vi "Plot init properties.vi"(5 "First call? (init)":bool, 7 "# plots":i32=2, 8 "error in (no error)":errorcluster, 11 "Refs":T1) -> (0 "error out":errorcluster, 3 "Refs (dup)":T1)   [LabVIEW 2021, in "RocketPlot.lvlib"]
uses:
  RocketPlot.lvlib
  TypeDefs/Plot UI references.ctl
  Classes/RocketPlotHandle/RocketPlotHandle.lvclass
  <userlib>/bjustice/TipStripOOPanel/Classes/TipPanelHandle/TipPanelHandle.lvclass
  TypeDefs/Plot top row.ctl
  TypeDefs/plot load data V2.ctl
  TypeDefs/plot properties V2.ctl
  TypeDefs/plot attributes V2.ctl
  TypeDefs/Plot scale axis properties.ctl
  TypeDefs/Plot general properties.ctl
  <vilib>/Utility/miscctls.llb/LVPositionTypeDef.ctl
  <vilib>/Utility/miscctls.llb/LVPointTypeDef.ctl
  <vilib>/Utility/colorconv.llb/RGB to Color.vi
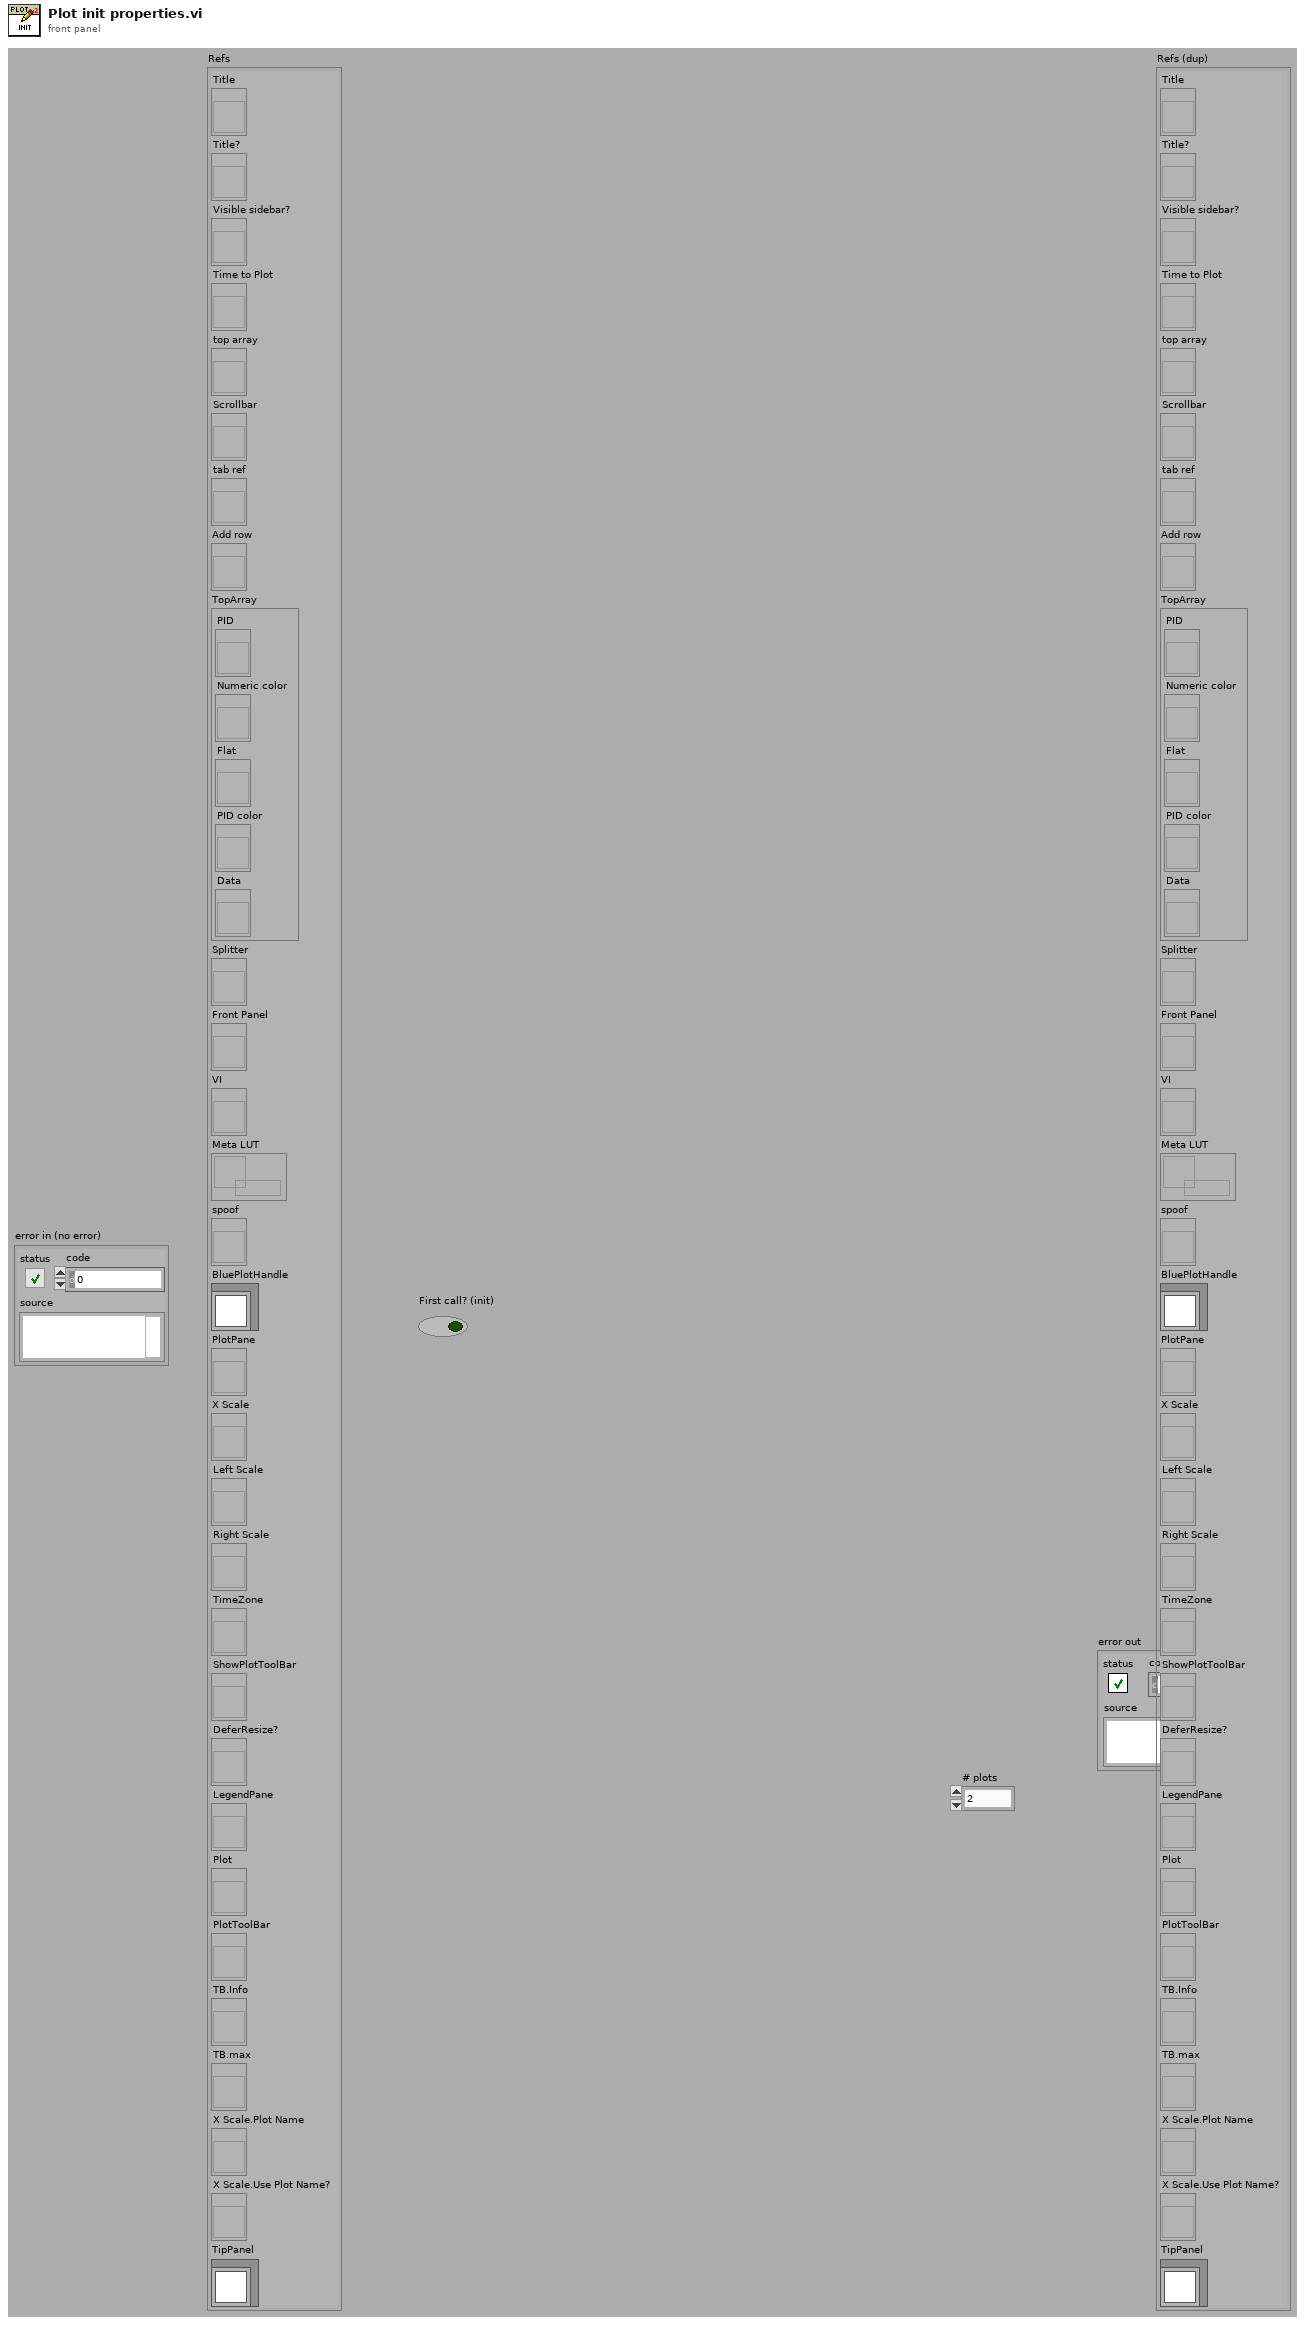
[diagram p1: front panel]
types:
  T1 = typedef "RocketPlot.lvlib/Plot UI references.ctl" = cluster{"Title":refnum<vi>, "Title?":refnum<vi>, "Visible sidebar?":refnum<vi>, "Time to Plot":refnum<vi>, "top array":refnum<vi>, "Scrollbar":refnum<vi>, "tab ref":refnum<vi>, "Add row":refnum<vi>, "TopArray":cluster{"PID":refnum<vi>, "Numeric color":refnum<vi>, "Flat":refnum<vi>, "PID color":refnum<vi>, "Data":refnum<vi>}, "Splitter":refnum<vi>, "Front Panel":refnum<vi>, "VI":refnum<vi>, "Meta LUT":refnum<data-value>, "spoof":refnum<vi>, "BluePlotHandle":refnum<class "RocketPlotHandle.lvclass">, "PlotPane":refnum<vi>, "X Scale":refnum<vi>, "Left Scale":refnum<vi>, "Right Scale":refnum<vi>, "TimeZone":refnum<vi>, "ShowPlotToolBar":refnum<vi>, "DeferResize?":refnum<vi>, "LegendPane":refnum<vi>, "Plot":refnum<vi>, "PlotToolBar":refnum<vi>, "TB.Info":refnum<vi>, "TB.max":refnum<vi>, "X Scale.Plot Name":refnum<vi>, "X Scale.Use Plot Name?":refnum<vi>, "TipPanel":refnum<class "TipPanelHandle.lvclass">}
  T2 = typedef "RocketPlot.lvlib/plot load data V2.ctl" = cluster{"plots":T3[], "X-axis":T5, "Y-axes":T5[], "General":T6}
  T3 = typedef "RocketPlot.lvlib/plot properties V2.ctl" = cluster{"attributes":T4, "Numeric":dbl, "Flatline?":bool}
  T4 = typedef "RocketPlot.lvlib/plot attributes V2.ctl" = cluster{"Plot Color":u32, "Point Style":u8, "Line Style":u8, "Plot Interpolation":u8, "Line Width":u8, "Bar Plot Style":u8, "Fill To":i16, "X Scale Index":u32, "Y Scale Index":u32, "Anti-aliased":bool, "Label Format":u8, "Digital Transition Type":u8, "Digital Transition Location":u8, "Digital Line Style":u8, "Fill/Point Color":u32, "Plot Name":string, "Visible":bool}
  T5 = typedef "RocketPlot.lvlib/Plot scale axis properties.ctl" = cluster{"Name Label.Text":string, "Style":u8, "Tick Colors:Minor Tick Color":u32, "Tick Colors:Tick Color":u32, "Marker Colors:Text Color":u32, "Grid Colors:Major Color":u32, "Grid Colors:Minor Color":u32, "Mapping Mode":u8, "Flipped":bool, "Name Label.Visible":bool, "Name Label.Text Colors:Text Color":u32, "Scale Fit":u8, "Range:Maximum":dbl, "Range:Minimum":dbl, "Offset and Multiplier:Multiplier":dbl, "Offset and Multiplier:Offset":dbl, "Name Label.Font:Size":u32, "Marker.Font:Size":u32, "Uniform Marker Spacing?":bool, "Format String":string}
  T6 = typedef "RocketPlot.lvlib/Plot general properties.ctl" = cluster{"Title":string, "Time to Plot":dbl, "Title.Visible":bool, "Sidebar.Visible":bool, "Plot Area:Colors:BG Color":u32, "X Scale.Plot Name":string, "X Scale.Use Plot Name":bool}
  T7 = typedef "LVPointTypeDef.ctl" = cluster{"Horizontal":i16, "Vertical":i16}
  T8 = typedef "LVPositionTypeDef.ctl" = cluster{"Left":i32, "Top":i32}
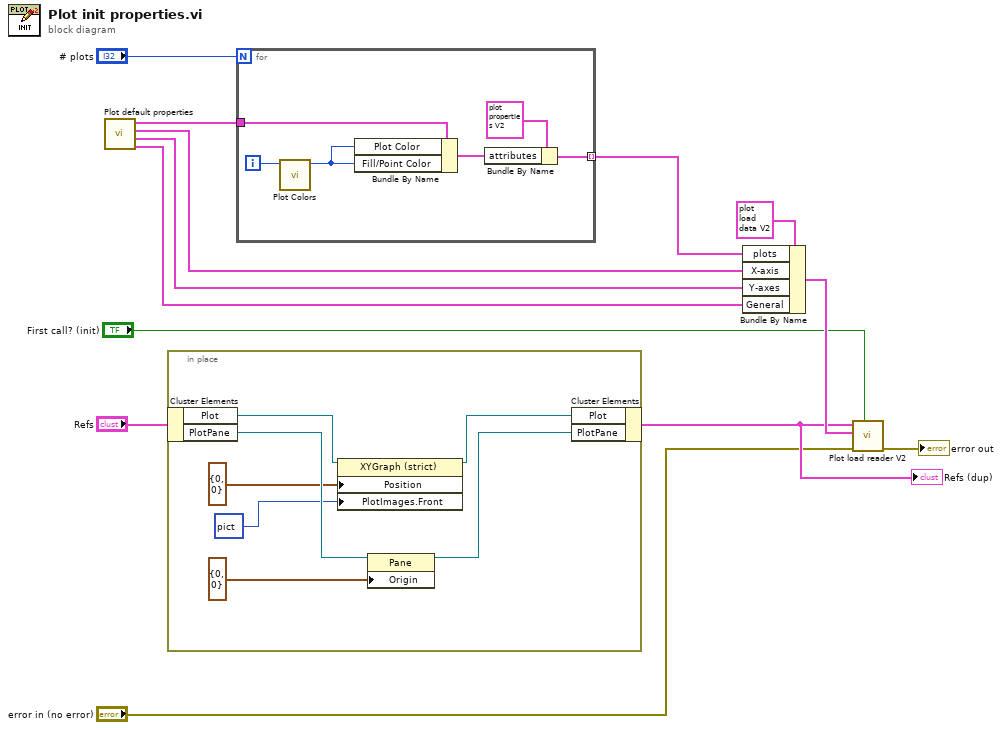
[diagram p0: block diagram]
diagram:
  n1 = call "Plot default properties.vi"() -> ("General"=w12:T6, "Default Y-axes"=w11:T5[], "Default X-axis"=w10:T5, "Default Attributes"=w8:T4)  [unwired: 7 in, 1 out]
  n2 = in-place {
    n3 = in-place-cluster #1("Refs") -> ("Plot"=w20:refnum<vi>, "PlotPane"=w17:refnum<vi>)
    n4 = property class="XYGraph (strict)"(reference=w20, "Position"=T8 {"Left"=0, "Top"=0}, "PlotImages.Front"=picture data[5B] ("Plot Images:Front")) -> (reference out=w19:refnum<vi>)  [unwired: 1 in, 1 out]
    n5 = property class="Pane"(reference=w17, "Origin"=T7 {"Horizontal"=0, "Vertical"=0}) -> (reference out=w16:refnum<vi>)  [unwired: 1 in, 1 out]
    n6 = in-place-cluster #1("Plot"=w19, "PlotPane"=w16) -> (w3:T1)
  }
  "Refs (dup)" <- w3
  n7 = for {
    N: "# plots" -> [_]
    tunnel: w8 -> [w24]
    tunnel: [w21] -> w7 mode=indexing
    i -> [w25]
    n8 = call "Plot Colors.vi"("Plot Index"=w25) -> ("Color Box"=w26:u32)  [unwired: 10 in]
    n9 = Bundle By Name(cluster=w24, "Plot Color"=w26, "Fill/Point Color"=w26) -> (w22:T4)
    n10 = Bundle By Name(cluster=T3 {"attributes"={"Plot Color"=0, "Point Style"=0, "Line Style"=0, "Plot Interpolation"=0, "Line Width"=0, "Bar Plot Style"=0, "Fill To"=0, "X Scale Index"=0, "Y Scale Index"=0, "Anti-aliased"=FALSE, "Label Format"=0, "Digital Transition Type"=0, "Digital Transition Location"=0, "Digital Line Style"=0, "Fill/Point Color"=0, "Plot Name"="", "Visible"=FALSE}, "Numeric"=0.0, "Flatline?"=FALSE} ("Cluster"), "attributes"=w22) -> (w21:T3)
  }
  n11 = Bundle By Name(cluster=T2 {"plots"=[], "X-axis"={"Name Label.Text"="", "Style"=0, "Tick Colors:Minor Tick Color"=0, "Tick Colors:Tick Color"=0, "Marker Colors:Text Color"=0, "Grid Colors:Major Color"=0, "Grid Colors:Minor Color"=0, "Mapping Mode"=0, "Flipped"=FALSE, "Name Label.Visible"=FALSE, "Name Label.Text Colors:Text Color"=0, "Scale Fit"=0, "Range:Maximum"=0.0, "Range:Minimum"=0.0, "Offset and Multiplier:Multiplier"=0.0, "Offset and Multiplier:Offset"=0.0, "Name Label.Font:Size"=0, "Marker.Font:Size"=0, "Uniform Marker Spacing?"=TRUE, "Format String"=""}, "Y-axes"=[], "General"={"Title"="", "Time to Plot"=1800.0, "Title.Visible"=FALSE, "Sidebar.Visible"=FALSE, "Plot Area:Colors:BG Color"=0, "X Scale.Plot Name"="", "X Scale.Use Plot Name"=FALSE}} ("Plot config"), "plots"=w7, "X-axis"=w10, "Y-axes"=w11, "General"=w12) -> (w6:T2)
  n12 = call "Plot load reader V2.vi"("First call? (init)"="First call? (init)", "error in (no error)"="error in (no error)", "Plot config"=w6, "Refs"=w3) -> ("error out"=→"error out":errorcluster)  [unwired: 7 in]
